vi "SystemDataDestroy.vi"(8 "error in (no error)":errorcluster) -> (0 "error out":errorcluster)   [LabVIEW 2014, in "SystemData.lvclass"]
uses:
  SystemData.lvclass
  Singleton.lvclass/Destructor.vi
  Singleton.lvclass/Constructor.vi
  Singleton.lvclass/Singleton.lvclass
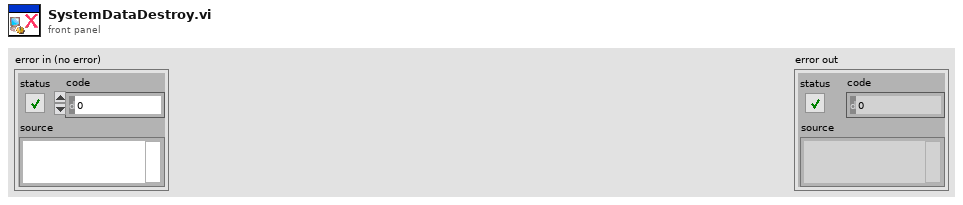
[diagram p1: front panel]
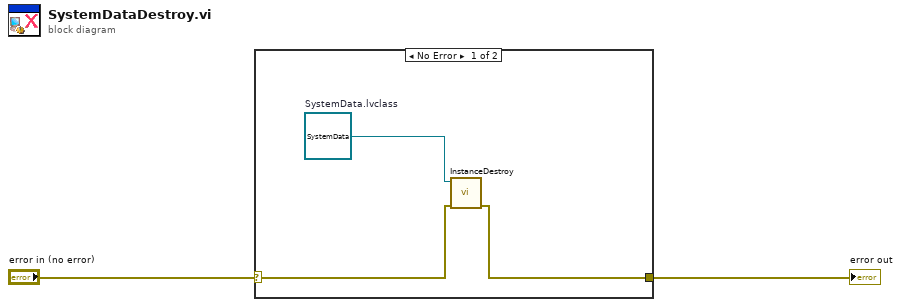
[diagram p0: block diagram]
diagram:
  n1 = case shown="No Error" "error in (no error)" {
    selector: "error in (no error)" -> [w5 w6]
    tunnel: [w4 w6] -> w1
    frame No Error {
      w3 = refnum<class "SystemData.lvclass"> refnum  # SystemData.lvclass
      n2 = call "InstanceDestroy.vi"("error in (no error)"=w5, "Singleton.lvclass In"=w3) -> ("error out"=w4:errorcluster)  [unwired: 8 in, 1 out]
    }
    frame Error {
    }
  }
  "error out" <- w1
